vi "SetParameters.vi"(0 "Camera Reference in":refnum<k24>, 1 "error in (no error)":errorcluster, 2 "2D Exposure Mode (Timed Auto HDR Flash)":enum16{"Timed", "Auto", "HDR", "Flash"}(ring), 3 "2D Exposure Time (0.1-999)":dbl=0.1 min=0.1 max=999.0 step=0.1, 4 "2D Gray Value":i32 min=0 max=255 step=1, 5 "2D Auto-Exposure ROI (x, y, width, height)":T2, 6 "2D Tone Mapping":bool, 7 "2D HDR Exposure Count":i32=1 min=1 max=5 step=1, 8 "2D HDR Exposure Sequence":T1={"Exposure 1"=0.1, "Exposure 2"=0.1, "Exposure 3"=0.1, "Exposure 4"=0.1, "Exposure 5"=0.1} {"Exposure 5" min=0.1 max=999.0; "Exposure 4" min=0.1 max=999.0; "Exposure 3" min=0.1 max=999.0; "Exposure 2" min=0.1 max=999.0; "Exposure 1" min=0.1 max=999.0}, 9 "3D Exposure Multiplier":i8=1 min=1 max=3 step=1, 10 "3D Exposure Sequence (value 0.1-99)":T3={"Exposure 1"=0.1, "Exposure 2"=0.1, "Exposure 3"=0.1} {"Exposure 3" min=0.1 max=99.0; "Exposure 2" min=0.1 max=99.0; "Exposure 1" min=0.1 max=99.0}, 11 "3D Gain (0-16)":dbl, 12 "Depth Range (lower upper)":cluster{"lower":i32, "upper":i32}, 13 "ROI (x, y, width, height)":T2, 16 "PointCloudSurfaceSmoothing (Off Weak Normal Strong)":u8(ring) items=["Off", "Weak", "Normal", "Strong"], 17 "PointCloudNoiseRemoval (Off Weak Normal Strong)":u8(ring) items=["Off", "Weak", "Normal", "Strong"], 18 "PointCloudOutlierRemoval (Off Weak Normal Strong)":u8(ring) items=["Off", "Weak", "Normal", "Strong"], 19 "Stripe Contrast Thresold (0-100)":i32 min=0 max=100 step=1) -> (14 "Camera Reference out":refnum<k24>, 15 "error out":errorcluster)   [LabVIEW 2023]
uses:
  C:/Mech-Mind/Mech-Eye SDK-2.5.0-c1-dev-01-17/API/dll/net48/MechEyeApiNet.dll
  dll/net48/MechEyeApiNet.dll
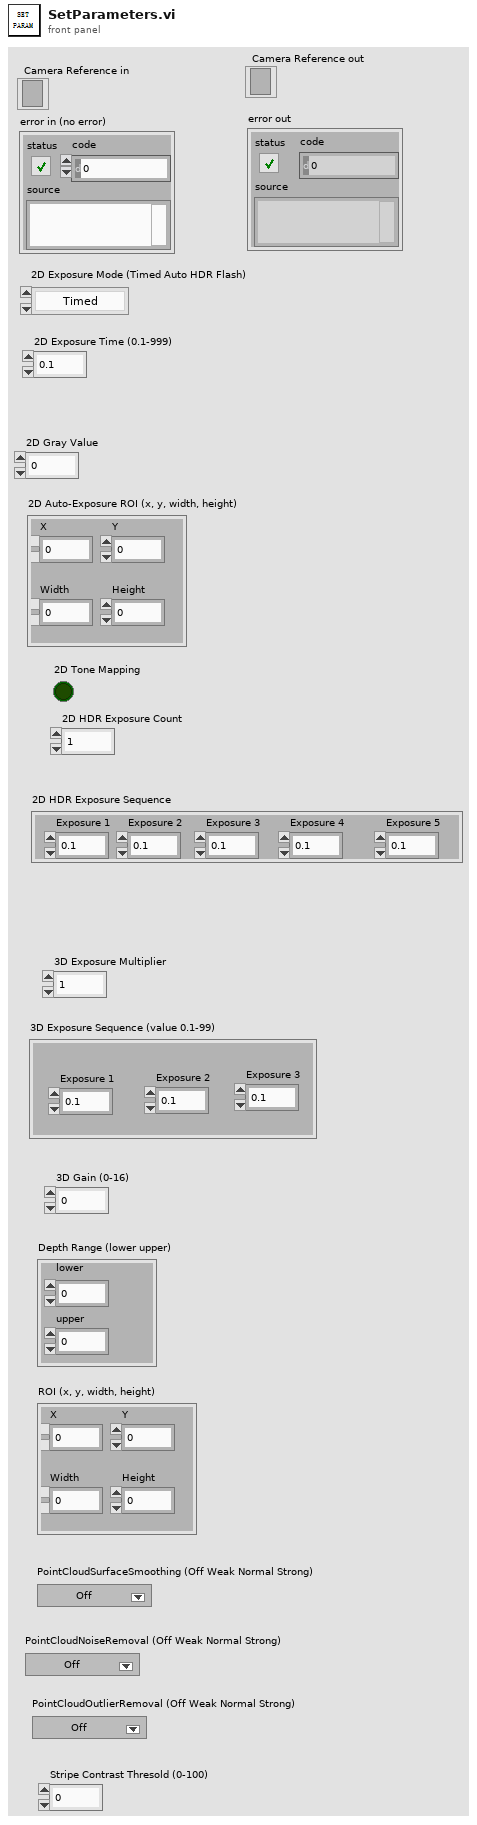
[diagram p1: front panel]
types:
  T1 = cluster{"Exposure 1":dbl, "Exposure 2":dbl, "Exposure 3":dbl, "Exposure 4":dbl, "Exposure 5":dbl}
  T2 = cluster{"X":i32, "Y":i32, "Width":i32, "Height":i32}
  T3 = cluster{"Exposure 1":dbl, "Exposure 2":dbl, "Exposure 3":dbl}
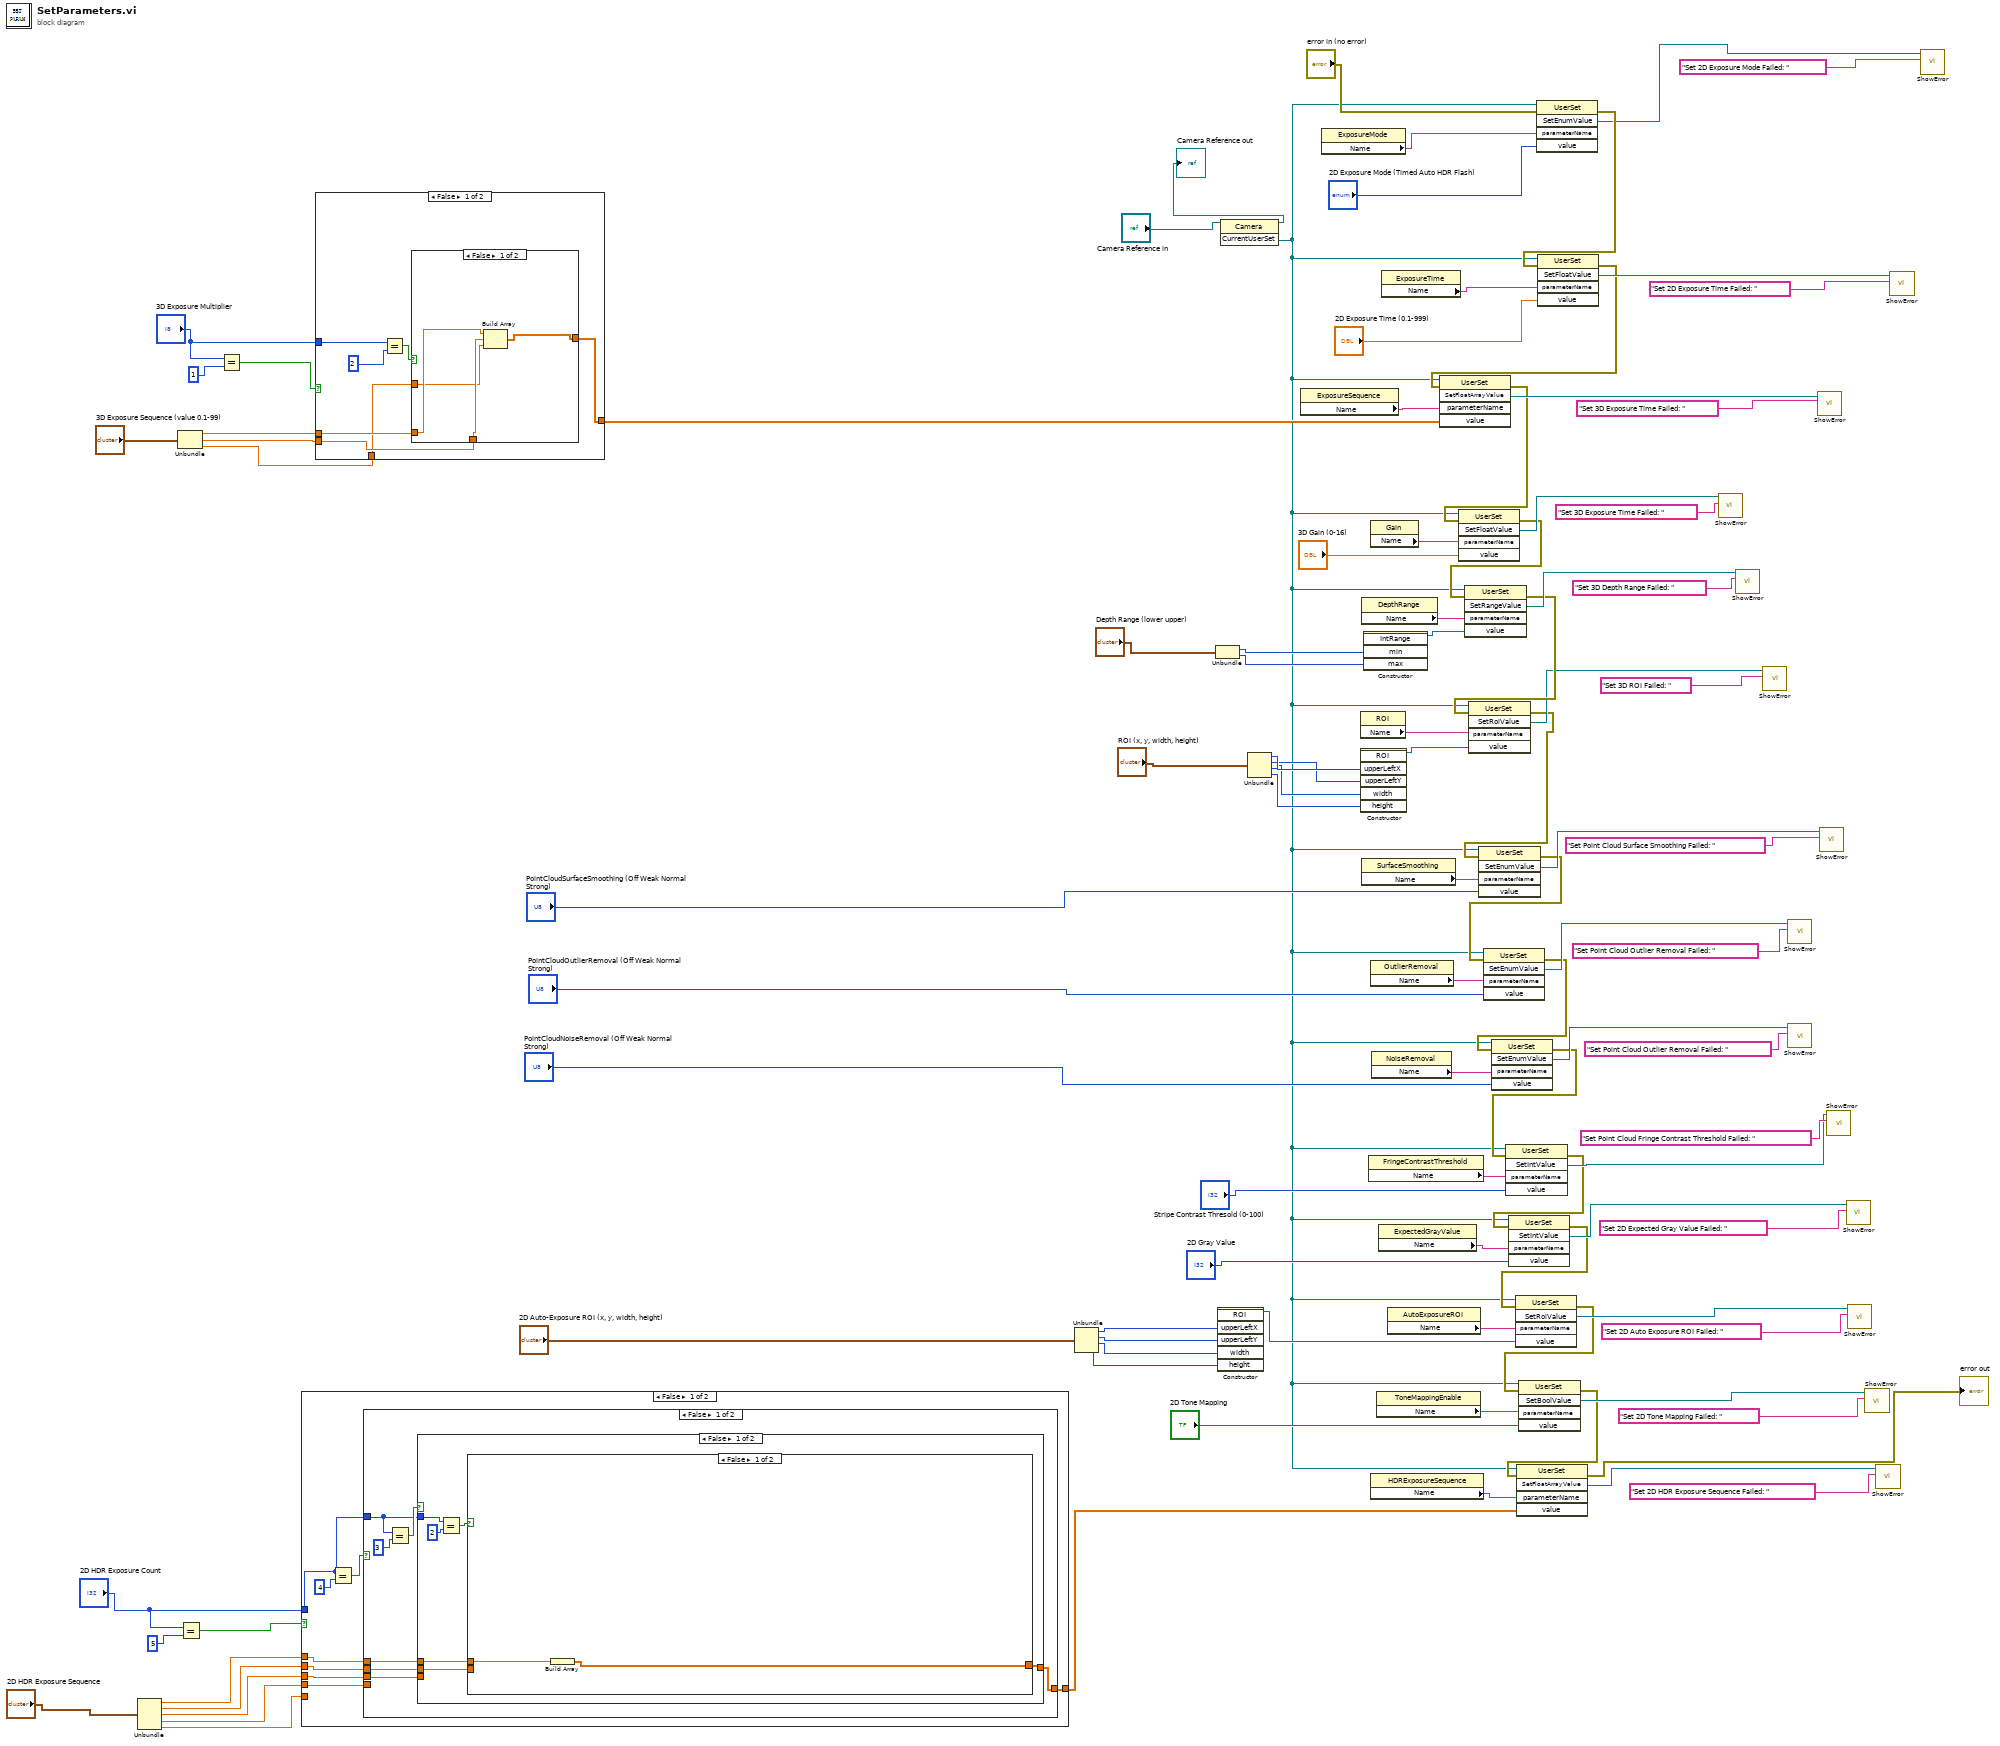
[diagram p0: block diagram]
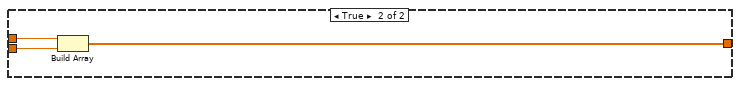
[diagram p2: hidden frame]
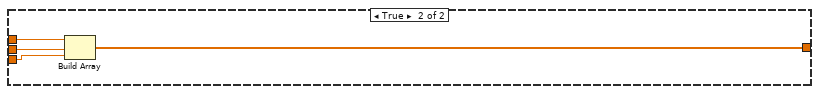
[diagram p3: hidden frame]
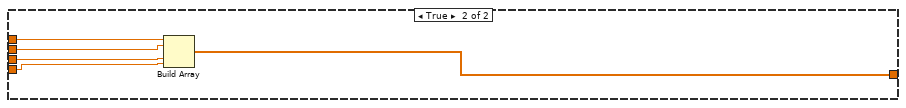
[diagram p4: hidden frame]
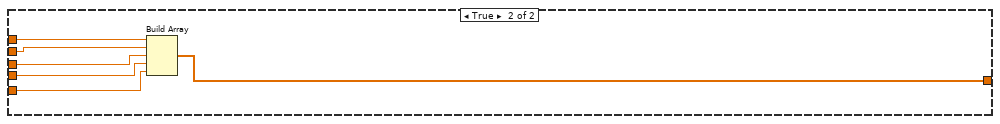
[diagram p5: hidden frame]
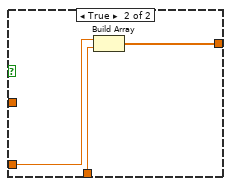
[diagram p6: hidden frame]
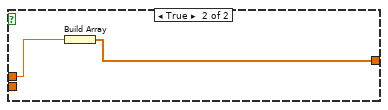
[diagram p7: hidden frame]
diagram:
  n1 = Unbundle("2D HDR Exposure Sequence") -> ("Exposure 1"=w13:dbl, "Exposure 2"=w12:dbl, "Exposure 3"=w11:dbl, "Exposure 4"=w6:dbl, "Exposure 5"=w5:dbl)
  n2 = Unbundle("3D Exposure Sequence (value 0.1-99)") -> ("Exposure 1"=w44:dbl, "Exposure 2"=w43:dbl, "Exposure 3"=w42:dbl)
  n3 = Equal?(x="2D HDR Exposure Count", y=5) -> (x = y?=w9:bool)
  n4 = Equal?(x="3D Exposure Multiplier", y=1) -> (x = y?=w39:bool)
  n5 = case shown="False" w9 {
    tunnel: w13 -> [w109 w144]
    tunnel: w12 -> [w108 w142]
    tunnel: w11 -> [w107 w141]
    tunnel: [w105 w143] -> w4
    tunnel: "2D HDR Exposure Count" -> [w104 _]
    tunnel: w6 -> [w106 w140]
    tunnel: w5 -> [_ w139]
    frame False {
      n6 = Equal?(x=w104, y=4) -> (x = y?=w110:bool)
      n7 = case shown="False" w110 {
        tunnel: w109 -> [w116 w138]
        tunnel: w108 -> [w115 w137]
        tunnel: w107 -> [w114 w136]
        tunnel: w106 -> [_ w135]
        tunnel: [w113 w134] -> w105
        tunnel: w104 -> [w112 _]
        frame False {
          n8 = Equal?(x=w112, y=3) -> (x = y?=w117:bool)
          n9 = case shown="False" w117 {
            tunnel: w116 -> [w121 w133]
            tunnel: w115 -> [w120 w132]
            tunnel: w114 -> [_ w131]
            tunnel: [w119 w130] -> w113
            tunnel: w112 -> [w124 _]
            frame False {
              n10 = Equal?(x=w124, y=2) -> (x = y?=w122:bool)
              n11 = case shown="False" w122 {
                tunnel: w121 -> [w126 w129]
                tunnel: w120 -> [_ w128]
                tunnel: [w125 w127] -> w119
                frame False {
                  n12 = Build Array(w126) -> (w125:dbl[])
                }
                frame True {
                  n13 = Build Array(w129, w128) -> (w127:dbl[])
                }
              }
            }
            frame True {
              n14 = Build Array(w133, w132, w131) -> (w130:dbl[])
            }
          }
        }
        frame True {
          n15 = Build Array(w138, w137, w136, w135) -> (w134:dbl[])
        }
      }
    }
    frame True {
      n16 = Build Array(w144, w142, w141, w140, w139) -> (w143:dbl[])
    }
  }
  n17 = case shown="False" w39 {
    tunnel: w44 -> [w148 w160]
    tunnel: w43 -> [w147 _]
    tunnel: w42 -> [w145 _]
    tunnel: [w146 w159] -> w41
    tunnel: "3D Exposure Multiplier" -> [w151 _]
    frame False {
      n18 = Equal?(x=w151, y=2) -> (x = y?=w149:bool)
      n19 = case shown="False" w149 {
        tunnel: w148 -> [w155 w158]
        tunnel: w147 -> [w154 w157]
        tunnel: [w152 w156] -> w146
        tunnel: w145 -> [w153 _]
        frame False {
          n20 = Build Array(w155, w154, w153) -> (w152:dbl[])
        }
        frame True {
          n21 = Build Array(w158, w157) -> (w156:dbl[])
        }
      }
    }
    frame True {
      n22 = Build Array(w160) -> (w159:dbl[])
    }
  }
  n23 = Unbundle("2D Auto-Exposure ROI (x, y, width, height)") -> ("X"=w31:i32, "Y"=w30:i32, "Width"=w29:i32, "Height"=w28:i32)
  n24 = Unbundle("Depth Range (lower upper)") -> ("lower"=w51:i32, "upper"=w50:i32)
  n25 = constructor class="ROI"("upperLeftX"=w31, "upperLeftY"=w30, "width"=w29, "height"=w28) -> (reference out=w27:refnum<k24>)  [unwired: 3 in, 6 out]
  n26 = invoke class="Camera" method="CurrentUserSet"(reference="Camera Reference in") -> (reference out=→"Camera Reference out":refnum<k24>, "CurrentUserSet"=w15:refnum<k24>)  [unwired: 2 in, 1 out]
  n27 = Unbundle("ROI (x, y, width, height)") -> ("X"=w56:i32, "Y"=w55:i32, "Width"=w54:i32, "Height"=w53:i32)
  n28 = property class="ExposureSequence"() -> ("Name"=w94:string)  [unwired: 2 in, 2 out]
  n29 = property class="ExposureMode"() -> ("Name"=w96:string)  [unwired: 2 in, 2 out]
  n30 = property class="ROI"() -> ("Name"=w81:string)  [unwired: 2 in, 2 out]
  n31 = constructor class="ROI"("upperLeftX"=w56, "upperLeftY"=w55, "width"=w54, "height"=w53) -> (reference out=w80:refnum<k24>)  [unwired: 3 in, 6 out]
  n32 = property class="DepthRange"() -> ("Name"=w88:string)  [unwired: 2 in, 2 out]
  n33 = property class="SurfaceSmoothing"() -> ("Name"=w78:string)  [unwired: 2 in, 2 out]
  n34 = constructor class="IntRange"("min"=w51, "max"=w50) -> (reference out=w87:refnum<k24>)  [unwired: 3 in, 4 out]
  n35 = property class="FringeContrastThreshold"() -> ("Name"=w61:string)  [unwired: 2 in, 2 out]
  n36 = property class="OutlierRemoval"() -> ("Name"=w73:string)  [unwired: 2 in, 2 out]
  n37 = property class="Gain"() -> ("Name"=w91:string)  [unwired: 2 in, 2 out]
  n38 = property class="HDRExposureSequence"() -> ("Name"=w14:string)  [unwired: 2 in, 2 out]
  n39 = property class="NoiseRemoval"() -> ("Name"=w70:string)  [unwired: 2 in, 2 out]
  n40 = property class="ToneMappingEnable"() -> ("Name"=w23:string)  [unwired: 2 in, 2 out]
  n41 = property class="ExpectedGrayValue"() -> ("Name"=w36:string)  [unwired: 2 in, 2 out]
  n42 = property class="ExposureTime"() -> ("Name"=w95:string)  [unwired: 2 in, 2 out]
  n43 = property class="AutoExposureROI"() -> ("Name"=w24:string)  [unwired: 2 in, 2 out]
  n44 = invoke class="UserSet" method="SetEnumValue"(reference=w15, error in="error in (no error)", "parameterName"=w96, "value"="2D Exposure Mode (Timed Auto HDR Flash)") -> (error out=w102:errorcluster, "SetEnumValue"=w99:refnum<k24>)  [unwired: 1 in, 3 out]
  n45 = invoke class="UserSet" method="SetFloatValue"(reference=w15, error in=w102, "parameterName"=w95, "value"="2D Exposure Time (0.1-999)") -> (error out=w84:errorcluster, "SetFloatValue"=w98:refnum<k24>)  [unwired: 1 in, 3 out]
  n46 = invoke class="UserSet" method="SetFloatArrayValue"(reference=w15, error in=w84, "parameterName"=w94, "value"=w41) -> (error out=w83:errorcluster, "SetFloatArrayValue"=w92:refnum<k24>)  [unwired: 1 in, 3 out]
  n47 = invoke class="UserSet" method="SetFloatValue"(reference=w15, error in=w83, "parameterName"=w91, "value"="3D Gain (0-16)") -> (error out=w82:errorcluster, "SetFloatValue"=w89:refnum<k24>)  [unwired: 1 in, 3 out]
  n48 = invoke class="UserSet" method="SetRangeValue"(reference=w15, error in=w82, "parameterName"=w88, "value"=w87) -> (error out=w79:errorcluster, "SetRangeValue"=w85:refnum<k24>)  [unwired: 1 in, 3 out]
  n49 = invoke class="UserSet" method="SetRoiValue"(reference=w15, error in=w79, "parameterName"=w81, "value"=w80) -> (error out=w67:errorcluster, "SetRoiValue"=w76:refnum<k24>)  [unwired: 1 in, 3 out]
  n50 = invoke class="UserSet" method="SetEnumValue"(reference=w15, error in=w67, "parameterName"=w78, "value"="PointCloudSurfaceSmoothing (Off Weak Normal Strong)") -> (error out=w66:errorcluster, "SetEnumValue"=w74:refnum<k24>)  [unwired: 1 in, 3 out]
  n51 = invoke class="UserSet" method="SetEnumValue"(reference=w15, error in=w66, "parameterName"=w73, "value"="PointCloudOutlierRemoval (Off Weak Normal Strong)") -> (error out=w65:errorcluster, "SetEnumValue"=w71:refnum<k24>)  [unwired: 1 in, 3 out]
  n52 = invoke class="UserSet" method="SetEnumValue"(reference=w15, error in=w65, "parameterName"=w70, "value"="PointCloudNoiseRemoval (Off Weak Normal Strong)") -> (error out=w64:errorcluster, "SetEnumValue"=w68:refnum<k24>)  [unwired: 1 in, 3 out]
  n53 = invoke class="UserSet" method="SetIntValue"(reference=w15, error in=w64, "parameterName"=w61, "value"="Stripe Contrast Thresold (0-100)") -> (error out=w19:errorcluster, "SetIntValue"=w62:refnum<k24>)  [unwired: 1 in, 3 out]
  n54 = invoke class="UserSet" method="SetIntValue"(reference=w15, error in=w19, "parameterName"=w36, "value"="2D Gray Value") -> (error out=w18:errorcluster, "SetIntValue"=w33:refnum<k24>)  [unwired: 1 in, 3 out]
  n55 = invoke class="UserSet" method="SetRoiValue"(reference=w15, error in=w18, "parameterName"=w24, "value"=w27) -> (error out=w17:errorcluster, "SetRoiValue"=w25:refnum<k24>)  [unwired: 1 in, 3 out]
  n56 = invoke class="UserSet" method="SetBoolValue"(reference=w15, error in=w17, "parameterName"=w23, "value"="2D Tone Mapping") -> (error out=w16:errorcluster, "SetBoolValue"=w20:refnum<k24>)  [unwired: 1 in, 3 out]
  n57 = invoke class="UserSet" method="SetFloatArrayValue"(reference=w15, error in=w16, "parameterName"=w14, "value"=w4) -> (error out=→"error out":errorcluster, "SetFloatArrayValue"=w2:refnum<k24>)  [unwired: 1 in, 3 out]
  n58 = call "ShowError.vi"("String"="Set 3D Exposure Time Failed: ", "MMind.Eye.ErrorStatus"=w89) -> ()  [unwired: 10 in]
  n59 = call "ShowError.vi"("String"="Set 3D Depth Range Failed: ", "MMind.Eye.ErrorStatus"=w85) -> ()  [unwired: 10 in]
  n60 = call "ShowError.vi"("String"="Set 3D ROI Failed: ", "MMind.Eye.ErrorStatus"=w76) -> ()  [unwired: 10 in]
  n61 = call "ShowError.vi"("String"="Set Point Cloud Outlier Removal Failed: ", "MMind.Eye.ErrorStatus"=w71) -> ()  [unwired: 10 in]
  n62 = call "ShowError.vi"("String"="Set Point Cloud Outlier Removal Failed: ", "MMind.Eye.ErrorStatus"=w68) -> ()  [unwired: 10 in]
  n63 = call "ShowError.vi"("String"="Set 3D Exposure Time Failed: ", "MMind.Eye.ErrorStatus"=w92) -> ()  [unwired: 10 in]
  n64 = call "ShowError.vi"("String"="Set Point Cloud Surface Smoothing Failed: ", "MMind.Eye.ErrorStatus"=w74) -> ()  [unwired: 10 in]
  n65 = call "ShowError.vi"("String"="Set Point Cloud Fringe Contrast Threshold Failed: ", "MMind.Eye.ErrorStatus"=w62) -> ()  [unwired: 10 in]
  n66 = call "ShowError.vi"("String"="Set 2D Expected Gray Value Failed: ", "MMind.Eye.ErrorStatus"=w33) -> ()  [unwired: 10 in]
  n67 = call "ShowError.vi"("String"="Set 2D Auto Exposure ROI Failed: ", "MMind.Eye.ErrorStatus"=w25) -> ()  [unwired: 10 in]
  n68 = call "ShowError.vi"("String"="Set 2D Tone Mapping Failed: ", "MMind.Eye.ErrorStatus"=w20) -> ()  [unwired: 10 in]
  n69 = call "ShowError.vi"("String"="Set 2D HDR Exposure Sequence Failed: ", "MMind.Eye.ErrorStatus"=w2) -> ()  [unwired: 10 in]
  n70 = call "ShowError.vi"("String"="Set 2D Exposure Time Failed: ", "MMind.Eye.ErrorStatus"=w98) -> ()  [unwired: 10 in]
  n71 = call "ShowError.vi"("String"="Set 2D Exposure Mode Failed: ", "MMind.Eye.ErrorStatus"=w99) -> ()  [unwired: 10 in]
